vi "Write to DB.vi"(8 "error in (no error)":errorcluster, 10 "DB Record":T1 {"Balance" format="%.2f"; "Account" format="%05d"}, 11 "refnum":refnum<file>) -> (0 "error out":errorcluster, 3 "refnum out":refnum<file>)   [LabVIEW 2017]
uses:
  Type Definitions/DB Record.ctl
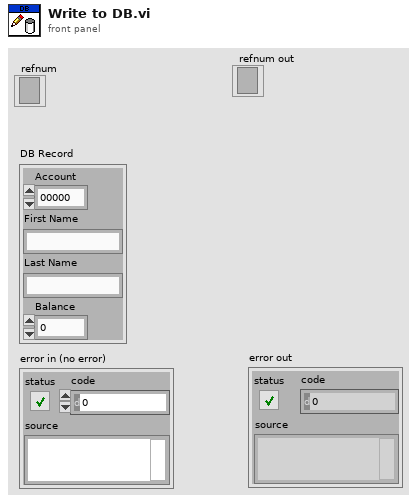
[diagram p1: front panel]
types:
  T1 = typedef "DB Record.ctl" = cluster{"Account":i32, "First Name":string, "Last Name":string, "Balance":fxp<+/-,64,35>}
  T2 = enum16{"open", "replace", "create", "open or create", "replace or create", "replace or create with confirmation"}
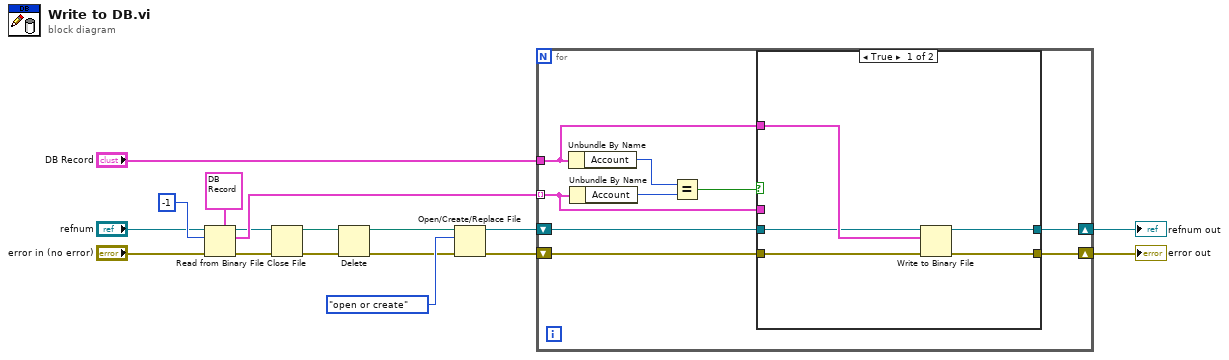
[diagram p0: block diagram]
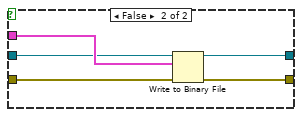
[diagram p2: hidden frame]
diagram:
  n1 = Read from Binary File(5:T1 {"Account"=0, "First Name"="", "Last Name"="", "Balance"=0.0} ("DB Record"), 8:"error in (no error)", 10:-1 ("count (1)"), 11:"refnum") -> (0:w10:errorcluster, 2:w16:T1[], 3:w3:refnum<file>)  [unwired: 2 in, 1 out]
  n2 = Close File(refnum=w3, error in=w10) -> (path=w2:path, error out=w4:errorcluster)
  n3 = Delete(path (use dialog)=w2, error in=w4) -> (deleted path=w1:path, error out=w5:errorcluster)  [unwired: 3 in, 1 out]
  n4 = Open/Create/Replace File(file path (use dialog)=w1, error in=w5, operation (0:open)=T2."open or create") -> (refnum out=w8:refnum<file>, error out=w9:errorcluster)  [unwired: 3 in, 1 out]
  n5 = for {
    tunnel: w16 -> [w22] mode=indexing
    tunnel: "DB Record" -> [w23]
    shift-right: [w21] -> w6
    shift-left: w8 -> [w19]
    shift-right: [w20] -> w7
    shift-left: w9 -> [w18]
    n6 = Unbundle By Name(w23) -> ("Account"=w26:i32)
    n7 = Unbundle By Name(w22) -> ("Account"=w25:i32)
    n8 = Equal?(x=w26, y=w25) -> (x = y?=w24:bool)
    n9 = case shown="True" w24 {
      tunnel: w18 -> [w31 w36]
      tunnel: w23 -> [w30 _]
      tunnel: w22 -> [_ w33]
      tunnel: [w29 w35] -> w21
      tunnel: [w28 w34] -> w20
      tunnel: w19 -> [w27 w32]
      frame True {
        n10 = Write to Binary File(file (use dialog)=w27, data=w30, error in=w31) -> (refnum out=w29:refnum<file>, error out=w28:errorcluster)  [unwired: 3 in, 1 out]
      }
      frame False {
        n11 = Write to Binary File(file (use dialog)=w32, data=w33, error in=w36) -> (refnum out=w35:refnum<file>, error out=w34:errorcluster)  [unwired: 3 in, 1 out]
      }
    }
  }
  "error out" <- w7
  "refnum out" <- w6
